vi "Configure Trigger Layer.vi"(0 "VISA resource name":refnum<visa-resource-name>, 1 "Trigger Source (0: Auto-Internal)":i32(ring) items=["Auto-Internal", "Bus", "Timer", "INT1", "INT2", "LAN", "EXT1", "EXT2", "EXT3", "EXT4", "EXT5", "EXT6", "EXT7", "EXT8", "EXT9", "EXT10", "EXT11", "EXT12", "EXT13", "EXT14"], 2 "Timer Trigger Interval (2E-5 seconds)":dbl=2e-05, 5 "Channel (0: Channel 1)":i32(ring) items=["Channel 1", "Channel 2"], 7 "Device Action (2: Both)":i32(ring)=2 items=["Acquire", "Transient", "Both"], 9 "Trigger Count (1)":i32=1, 11 "error in (no error)":errorcluster, 12 "LXI Triggers For Normal Trigger":bool[](array[boolean])=[TRUE, TRUE, TRUE, TRUE, TRUE, TRUE, TRUE, TRUE], 13 "Trigger Delay (0 second)":dbl, 14 "Trigger Bypass Mode (1: OFF)":i32(ring)=1 items=["Once", "Off"]) -> (4 "VISA resource name out":refnum<visa-resource-name>, 15 "error out":errorcluster)   [LabVIEW 2023, in "Agilent B2900 Series.lvlib"]
doc: "Configures trigger layer in ARM-Trigger model. B2900 supports the ARM-Trigger model described in 1999 SCPI Command Reference. The ARM-Trigger model shows independent event detection for the ARM and Trigger layers."
uses:
  Agilent B2900 Series.lvlib
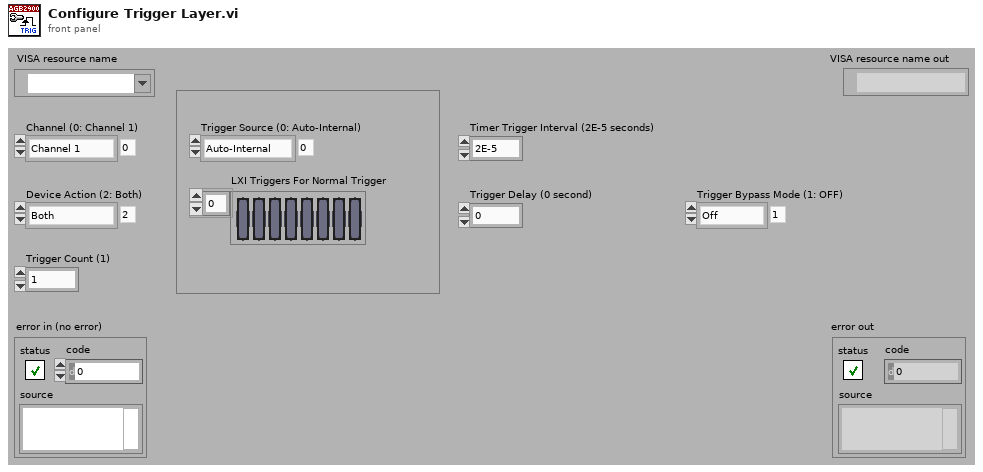
[diagram p1: front panel]
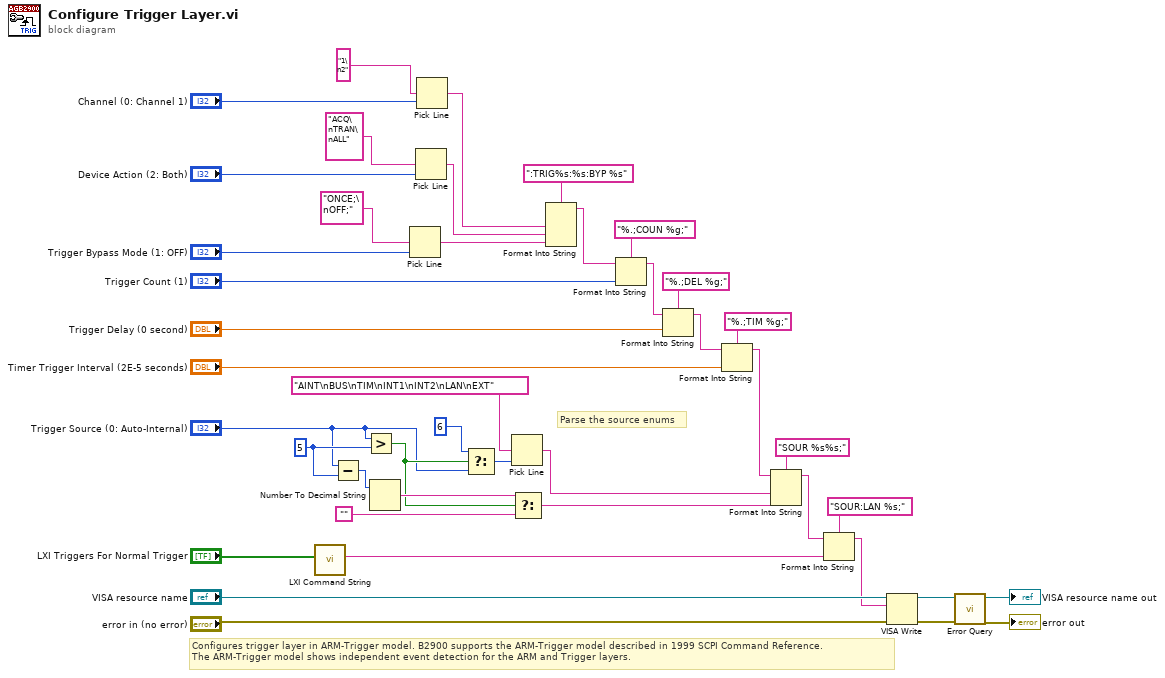
[diagram p0: block diagram]
diagram:
  w13 = 5 ("y")
  # "Configures trigger layer in ARM-Trigger model. B2900 supports the ARM-Trigger model described in 1999 SCPI Command Reference. \nThe ARM-Trigger model shows independent event detection for the ARM and Trigger layers."
  # "Parse the source enums"
  n1 = call "LXI Command String.vi"("LXI Triggers"="LXI Triggers For Normal Trigger") -> ("LXI Command String"=w15:string)  [unwired: 10 in]
  n2 = Subtract(x="Trigger Source (0: Auto-Internal)", y=w13) -> (x-y=w8:i32)
  n3 = Greater?(x="Trigger Source (0: Auto-Internal)", y=w13) -> (0:w9:bool)
  n4 = Number To Decimal String(number=w8) -> (decimal integer string=w11:string)  [unwired: 1 in]
  n5 = Pick Line(multi-line string="ONCE;\nOFF;", line index="Trigger Bypass Mode (1: OFF)") -> (output string=w21:string)  [unwired: 1 in]
  n6 = Pick Line(multi-line string="ACQ\nTRAN\nALL" ("string (\"\")"), line index="Device Action (2: Both)") -> (output string=w22:string)  [unwired: 1 in]
  n7 = Pick Line(multi-line string="1\n2" ("string (\"\")"), line index="Channel (0: Channel 1)") -> (output string=w23:string)  [unwired: 1 in]
  n8 = Select(t=6 ("f"), s=w9, f="Trigger Source (0: Auto-Internal)") -> (s? t:f=w10:i32)
  n9 = Pick Line(multi-line string="AINT\nBUS\nTIM\nINT1\nINT2\nLAN\nEXT", line index=w10) -> (output string=w5:string)  [unwired: 1 in]
  n10 = Select(t=w11, s=w9, f="") -> (s? t:f=w4:string)
  n11 = Format Into String(format string=":TRIG%s:%s:BYP %s" ("string (\"\")"), w23, w22, w21) -> (resulting string=w19:string)  [unwired: 2 in, 1 out]
  n12 = Format Into String(format string="%.;COUN %g;", initial string=w19, "Trigger Count (1)") -> (resulting string=w18:string)  [unwired: 1 in, 1 out]
  n13 = Format Into String(format string="%.;DEL %g;", initial string=w18, "Trigger Delay (0 second)") -> (resulting string=w17:string)  [unwired: 1 in, 1 out]
  n14 = Format Into String(format string="%.;TIM %g;", initial string=w17, "Timer Trigger Interval (2E-5 seconds)") -> (resulting string=w3:string)  [unwired: 1 in, 1 out]
  n15 = Format Into String(format string="SOUR %s%s;", initial string=w3, w5, w4) -> (resulting string=w2:string)  [unwired: 1 in, 1 out]
  n16 = Format Into String(format string="SOUR:LAN %s;", initial string=w2, w15) -> (resulting string=w1:string)  [unwired: 1 in, 1 out]
  n17 = VISA Write(VISA resource name="VISA resource name", write buffer=w1, error in (no error)="error in (no error)") -> (VISA resource name out=w31:refnum<visa-resource-name>, error out=w30:errorcluster)  [unwired: 1 out]
  n18 = call "Error Query.vi"("error in (no error)"=w30, "VISA resource name"=w31) -> ("error out"=→"error out":errorcluster, "VISA resource name out"=→"VISA resource name out":refnum<visa-resource-name>)  [unwired: 6 in, 2 out]
